vi "is hit.vi"(1 "Board with rocks":u32[][](array[numeric]), 2 "next row":i32, 3 "next column":i32, 4 "next orientation":i32) -> (0 "is hit":bool)   [LabVIEW 2019]
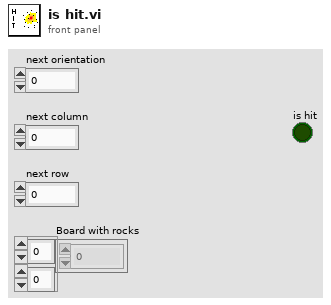
[diagram p1: front panel]
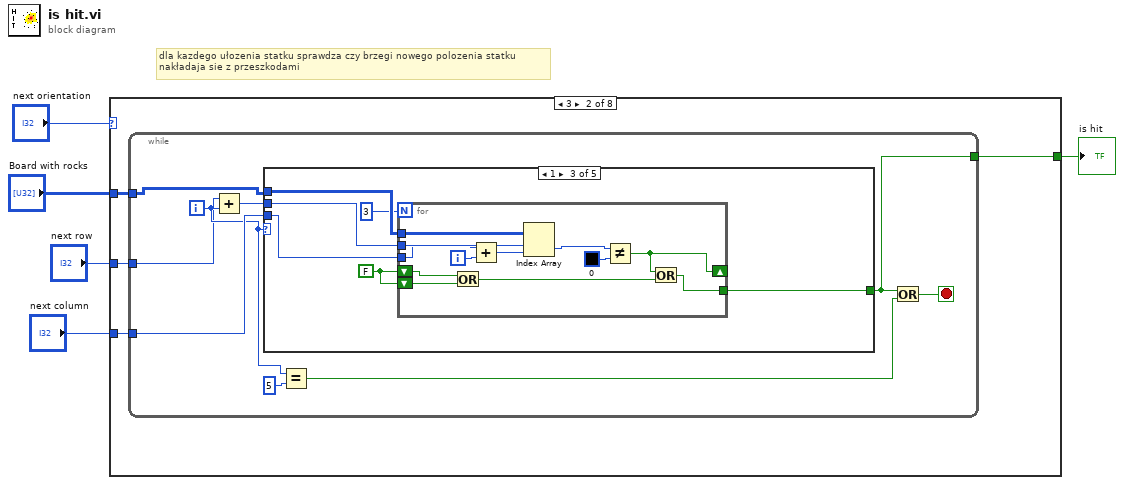
[diagram p0: block diagram]
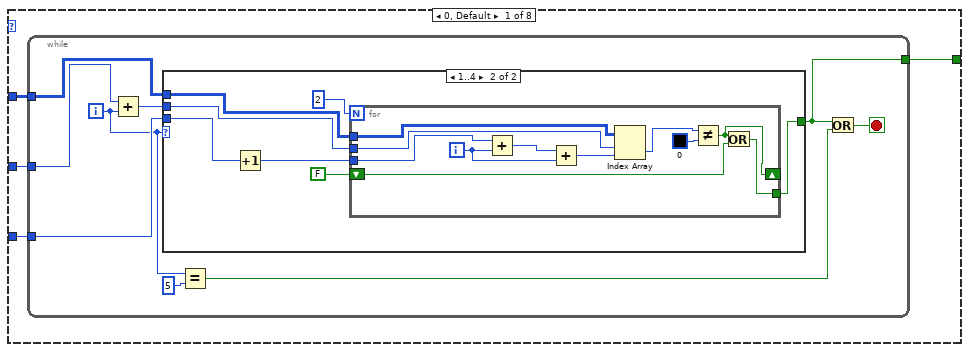
[diagram p2: hidden frame]
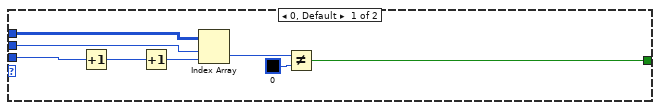
[diagram p3: hidden frame]
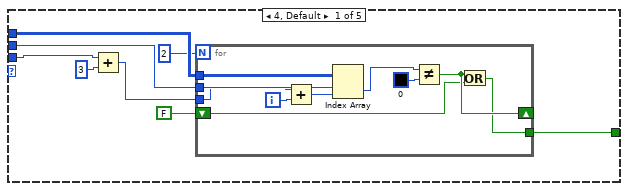
[diagram p4: hidden frame]
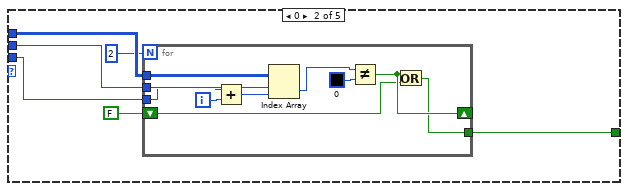
[diagram p5: hidden frame]
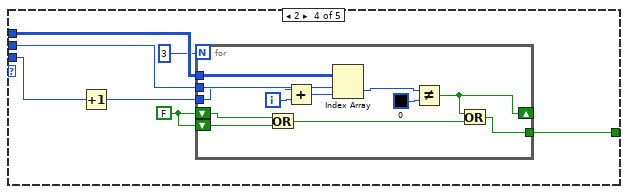
[diagram p6: hidden frame]
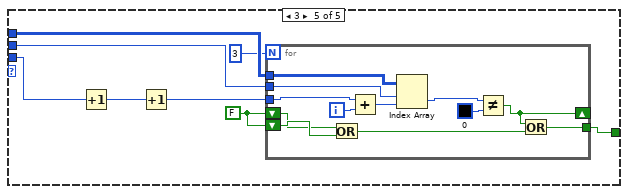
[diagram p7: hidden frame]
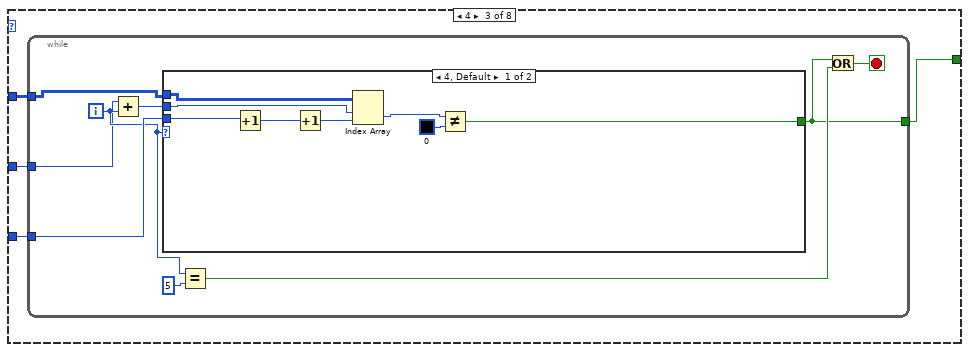
[diagram p8: hidden frame]
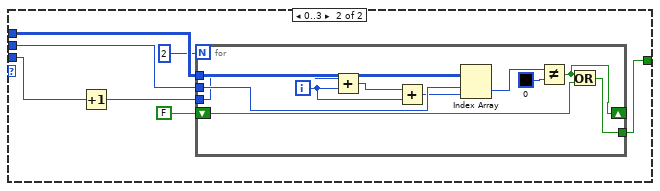
[diagram p9: hidden frame]
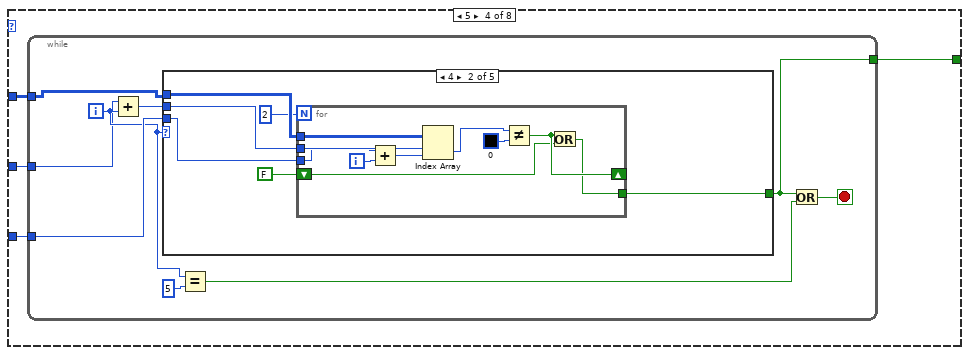
[diagram p10: hidden frame]
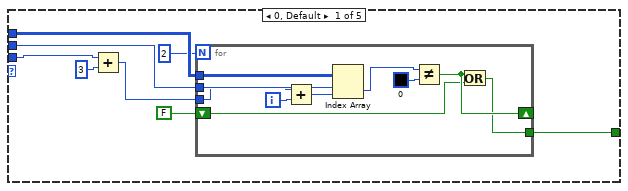
[diagram p11: hidden frame]
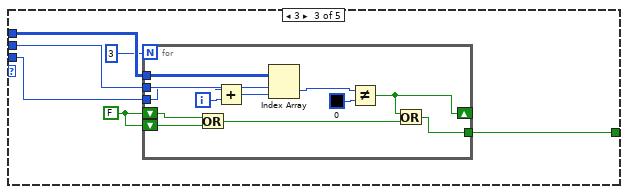
[diagram p12: hidden frame]
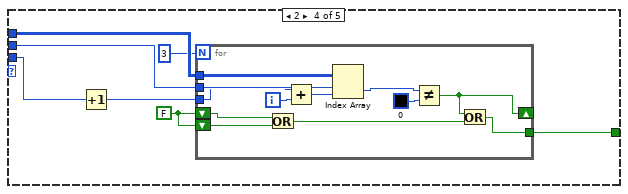
[diagram p13: hidden frame]
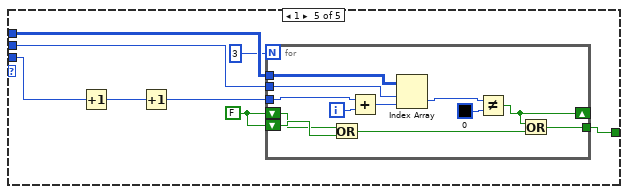
[diagram p14: hidden frame]
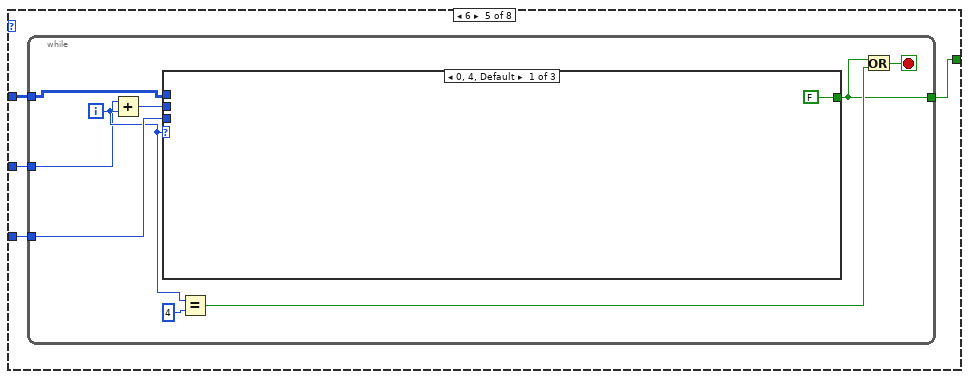
[diagram p15: hidden frame]
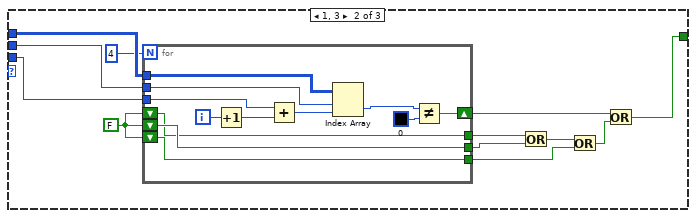
[diagram p16: hidden frame]
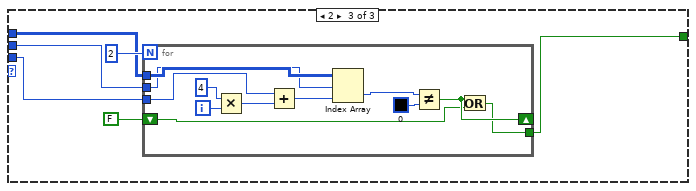
[diagram p17: hidden frame]
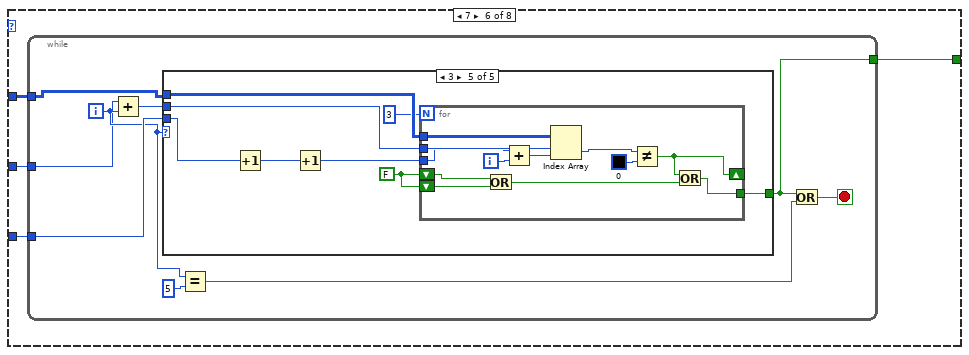
[diagram p18: hidden frame]
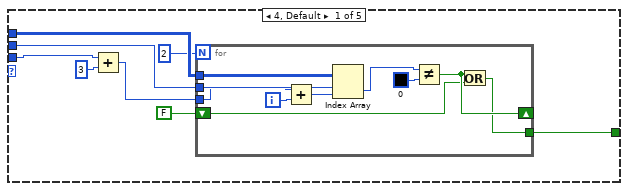
[diagram p19: hidden frame]
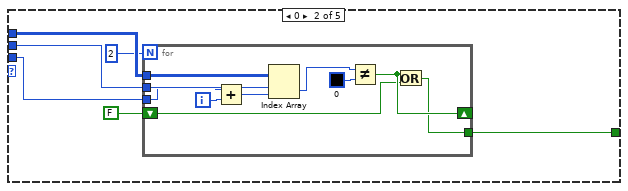
[diagram p20: hidden frame]
diagram:
  # "dla kazdego ułozenia statku sprawdza czy brzegi nowego polozenia statku \nnakładaja sie z przeszkodami"
  n1 = case shown="3" "next orientation" {
    tunnel: "next column" -> [w7 w46 w150 w189 w293 w349 w455 w557]
    tunnel: "next row" -> [w8 w47 w151 w190 w294 w350 w454 w558]
    tunnel: "Board with rocks" -> [w9 w48 w152 w191 w295 w351 w453 w559]
    tunnel: [w6 w45 w149 w188 w292 w348 w452 w556] -> w1
    frame 0, Default {
      n2 = while {
        tunnel: [w13] -> w6
        tunnel: w9 -> [w18]
        tunnel: w8 -> [w10]
        tunnel: w7 -> [w14]
        i -> [w12]
        stop <- w15 stop-if-true
        n3 = Add(x=w10, y=w12) -> (x+y=w11:i32)
        n4 = case shown="1..4" w12 {
          tunnel: w18 -> [w26 w33]
          tunnel: w11 -> [w25 w28]
          tunnel: w14 -> [w20 w30]
          tunnel: [w22 w27] -> w13
          frame 0, Default {
            n5 = Increment(x=w20) -> (x+1=w19:i32)
            n6 = Increment(x=w19) -> (x+1=w24:i32)
            n7 = Index Array(array=w26, index (row)=w25, index (col)=w24) -> (element=w21:u32)
            n8 = Not Equal?(x=w21, y=u32 0 ("Color Box")) -> (x != y?=w22:bool)
          }
          frame 1..4 {
            n9 = Increment(x=w30) -> (x+1=w29:i32)
            n10 = for {
              N: 2 -> [_]
              tunnel: w33 -> [w43]
              tunnel: w28 -> [w42]
              tunnel: w29 -> [w41]
              shift-right: [w36] -> _
              shift-left: FALSE -> [w35]
              tunnel: [w34] -> w27
              i -> [w38]
              n11 = Add(x=w41, y=w38) -> (x+y=w39:i32)
              n12 = Add(x=w39, y=w38) -> (x+y=w37:i32)
              n13 = Index Array(array=w43, index (row)=w42, index (col)=w37) -> (element=w40:u32)
              n14 = Not Equal?(x=w40, y=u32 0 ("Color Box")) -> (x != y?=w36:bool)
              n15 = Or(x=w36, y=w35) -> (x .or. y?=w34:bool)
            }
          }
        }
        n16 = Equal?(x=w12, y=5) -> (x = y?=w16:bool)
        n17 = Or(x=w13, y=w16) -> (x .or. y?=w15:bool)
      }
    }
    frame 3 {
      n18 = while {
        tunnel: [w52] -> w45
        tunnel: w48 -> [w57]
        tunnel: w47 -> [w49]
        tunnel: w46 -> [w53]
        i -> [w51]
        stop <- w54 stop-if-true
        n19 = Add(x=w49, y=w51) -> (x+y=w50:i32)
        n20 = case shown="1" w51 {
          tunnel: w57 -> [w65 w81 w97 w116 w136]
          tunnel: w50 -> [w62 w78 w95 w114 w134]
          tunnel: w53 -> [w60 w76 w93 w110 w131]
          tunnel: [w61 w77 w94 w113 w133] -> w52
          frame 4, Default {
            n21 = Add(x=w60, y=3) -> (x+y=w58:i32)
            n22 = for {
              N: 2 -> [_]
              tunnel: w65 -> [w74]
              tunnel: w62 -> [w73]
              tunnel: w58 -> [w72]
              shift-right: [w70] -> _
              shift-left: FALSE -> [w69]
              tunnel: [w68] -> w61
              i -> [w67]
              n23 = Add(x=w72, y=w67) -> (x+y=w66:i32)
              n24 = Index Array(array=w74, index (row)=w73, index (col)=w66) -> (element=w71:u32)
              n25 = Not Equal?(x=w71, y=u32 0 ("Color Box")) -> (x != y?=w70:bool)
              n26 = Or(x=w70, y=w69) -> (x .or. y?=w68:bool)
            }
          }
          frame 0 {
            n27 = for {
              N: 2 -> [_]
              tunnel: w81 -> [w90]
              tunnel: w78 -> [w89]
              tunnel: w76 -> [w88]
              shift-right: [w86] -> _
              shift-left: FALSE -> [w85]
              tunnel: [w84] -> w77
              i -> [w83]
              n28 = Add(x=w88, y=w83) -> (x+y=w82:i32)
              n29 = Index Array(array=w90, index (row)=w89, index (col)=w82) -> (element=w87:u32)
              n30 = Not Equal?(x=w87, y=u32 0 ("Color Box")) -> (x != y?=w86:bool)
              n31 = Or(x=w86, y=w85) -> (x .or. y?=w84:bool)
            }
          }
          frame 1 {
            w92 = FALSE
            n32 = for {
              N: 3 -> [_]
              tunnel: w97 -> [w108]
              tunnel: w95 -> [w107]
              tunnel: w93 -> [w106]
              shift-right: [w104] -> _
              shift-left: w92 -> [w99]
              tunnel: [w103] -> w94
              shift-left: w92 -> [w100]
              i -> [w102]
              n33 = Or(x=w99, y=w100) -> (x .or. y?=w98:bool)
              n34 = Add(x=w106, y=w102) -> (x+y=w101:i32)
              n35 = Index Array(array=w108, index (row)=w107, index (col)=w101) -> (element=w105:u32)
              n36 = Not Equal?(x=w105, y=u32 0 ("Color Box")) -> (x != y?=w104:bool)
              n37 = Or(x=w104, y=w98) -> (x .or. y?=w103:bool)
            }
          }
          frame 2 {
            w112 = FALSE
            n38 = Increment(x=w110) -> (x+1=w111:i32)
            n39 = for {
              N: 3 -> [_]
              tunnel: w116 -> [w127]
              tunnel: w114 -> [w126]
              tunnel: w111 -> [w125]
              shift-right: [w123] -> _
              shift-left: w112 -> [w118]
              tunnel: [w122] -> w113
              shift-left: w112 -> [w119]
              i -> [w121]
              n40 = Or(x=w118, y=w119) -> (x .or. y?=w117:bool)
              n41 = Add(x=w125, y=w121) -> (x+y=w120:i32)
              n42 = Index Array(array=w127, index (row)=w126, index (col)=w120) -> (element=w124:u32)
              n43 = Not Equal?(x=w124, y=u32 0 ("Color Box")) -> (x != y?=w123:bool)
              n44 = Or(x=w123, y=w117) -> (x .or. y?=w122:bool)
            }
          }
          frame 3 {
            w132 = FALSE
            n45 = Increment(x=w131) -> (x+1=w130:i32)
            n46 = Increment(x=w130) -> (x+1=w129:i32)
            n47 = for {
              N: 3 -> [_]
              tunnel: w136 -> [w147]
              tunnel: w134 -> [w146]
              tunnel: w129 -> [w145]
              shift-right: [w143] -> _
              shift-left: w132 -> [w138]
              tunnel: [w142] -> w133
              shift-left: w132 -> [w139]
              i -> [w141]
              n48 = Or(x=w138, y=w139) -> (x .or. y?=w137:bool)
              n49 = Add(x=w145, y=w141) -> (x+y=w140:i32)
              n50 = Index Array(array=w147, index (row)=w146, index (col)=w140) -> (element=w144:u32)
              n51 = Not Equal?(x=w144, y=u32 0 ("Color Box")) -> (x != y?=w143:bool)
              n52 = Or(x=w143, y=w137) -> (x .or. y?=w142:bool)
            }
          }
        }
        n53 = Equal?(x=w51, y=5) -> (x = y?=w55:bool)
        n54 = Or(x=w52, y=w55) -> (x .or. y?=w54:bool)
      }
    }
    frame 4 {
      n55 = while {
        tunnel: [w156] -> w149
        tunnel: w152 -> [w161]
        tunnel: w151 -> [w153]
        tunnel: w150 -> [w157]
        i -> [w155]
        stop <- w158 stop-if-true
        n56 = Add(x=w153, y=w155) -> (x+y=w154:i32)
        n57 = case shown="4, Default" w155 {
          tunnel: w161 -> [w169 w176]
          tunnel: w154 -> [w168 w171]
          tunnel: w157 -> [w163 w173]
          tunnel: [w165 w170] -> w156
          frame 4, Default {
            n58 = Increment(x=w163) -> (x+1=w162:i32)
            n59 = Increment(x=w162) -> (x+1=w167:i32)
            n60 = Index Array(array=w169, index (row)=w168, index (col)=w167) -> (element=w164:u32)
            n61 = Not Equal?(x=w164, y=u32 0 ("Color Box")) -> (x != y?=w165:bool)
          }
          frame 0..3 {
            n62 = Increment(x=w173) -> (x+1=w172:i32)
            n63 = for {
              N: 2 -> [_]
              tunnel: w176 -> [w186]
              tunnel: w171 -> [w185]
              tunnel: w172 -> [w184]
              shift-right: [w179] -> _
              shift-left: FALSE -> [w178]
              tunnel: [w177] -> w170
              i -> [w181]
              n64 = Add(x=w184, y=w181) -> (x+y=w182:i32)
              n65 = Add(x=w182, y=w181) -> (x+y=w180:i32)
              n66 = Index Array(array=w186, index (row)=w185, index (col)=w180) -> (element=w183:u32)
              n67 = Not Equal?(x=w183, y=u32 0 ("Color Box")) -> (x != y?=w179:bool)
              n68 = Or(x=w179, y=w178) -> (x .or. y?=w177:bool)
            }
          }
        }
        n69 = Equal?(x=w155, y=5) -> (x = y?=w159:bool)
        n70 = Or(x=w156, y=w159) -> (x .or. y?=w158:bool)
      }
    }
    frame 5 {
      n71 = while {
        tunnel: [w195] -> w188
        tunnel: w191 -> [w200]
        tunnel: w190 -> [w192]
        tunnel: w189 -> [w196]
        i -> [w194]
        stop <- w197 stop-if-true
        n72 = Add(x=w192, y=w194) -> (x+y=w193:i32)
        n73 = case shown="4" w194 {
          tunnel: w200 -> [w208 w224 w240 w259 w279]
          tunnel: w193 -> [w205 w221 w238 w257 w277]
          tunnel: w196 -> [w203 w219 w236 w253 w274]
          tunnel: [w204 w220 w237 w256 w276] -> w195
          frame 0, Default {
            n74 = Add(x=w203, y=3) -> (x+y=w201:i32)
            n75 = for {
              N: 2 -> [_]
              tunnel: w208 -> [w217]
              tunnel: w205 -> [w216]
              tunnel: w201 -> [w215]
              shift-right: [w213] -> _
              shift-left: FALSE -> [w212]
              tunnel: [w211] -> w204
              i -> [w210]
              n76 = Add(x=w215, y=w210) -> (x+y=w209:i32)
              n77 = Index Array(array=w217, index (row)=w216, index (col)=w209) -> (element=w214:u32)
              n78 = Not Equal?(x=w214, y=u32 0 ("Color Box")) -> (x != y?=w213:bool)
              n79 = Or(x=w213, y=w212) -> (x .or. y?=w211:bool)
            }
          }
          frame 4 {
            n80 = for {
              N: 2 -> [_]
              tunnel: w224 -> [w233]
              tunnel: w221 -> [w232]
              tunnel: w219 -> [w231]
              shift-right: [w229] -> _
              shift-left: FALSE -> [w228]
              tunnel: [w227] -> w220
              i -> [w226]
              n81 = Add(x=w231, y=w226) -> (x+y=w225:i32)
              n82 = Index Array(array=w233, index (row)=w232, index (col)=w225) -> (element=w230:u32)
              n83 = Not Equal?(x=w230, y=u32 0 ("Color Box")) -> (x != y?=w229:bool)
              n84 = Or(x=w229, y=w228) -> (x .or. y?=w227:bool)
            }
          }
          frame 3 {
            w235 = FALSE
            n85 = for {
              N: 3 -> [_]
              tunnel: w240 -> [w251]
              tunnel: w238 -> [w250]
              tunnel: w236 -> [w249]
              shift-right: [w247] -> _
              shift-left: w235 -> [w242]
              tunnel: [w246] -> w237
              shift-left: w235 -> [w243]
              i -> [w245]
              n86 = Or(x=w242, y=w243) -> (x .or. y?=w241:bool)
              n87 = Add(x=w249, y=w245) -> (x+y=w244:i32)
              n88 = Index Array(array=w251, index (row)=w250, index (col)=w244) -> (element=w248:u32)
              n89 = Not Equal?(x=w248, y=u32 0 ("Color Box")) -> (x != y?=w247:bool)
              n90 = Or(x=w247, y=w241) -> (x .or. y?=w246:bool)
            }
          }
          frame 2 {
            w255 = FALSE
            n91 = Increment(x=w253) -> (x+1=w254:i32)
            n92 = for {
              N: 3 -> [_]
              tunnel: w259 -> [w270]
              tunnel: w257 -> [w269]
              tunnel: w254 -> [w268]
              shift-right: [w266] -> _
              shift-left: w255 -> [w261]
              tunnel: [w265] -> w256
              shift-left: w255 -> [w262]
              i -> [w264]
              n93 = Or(x=w261, y=w262) -> (x .or. y?=w260:bool)
              n94 = Add(x=w268, y=w264) -> (x+y=w263:i32)
              n95 = Index Array(array=w270, index (row)=w269, index (col)=w263) -> (element=w267:u32)
              n96 = Not Equal?(x=w267, y=u32 0 ("Color Box")) -> (x != y?=w266:bool)
              n97 = Or(x=w266, y=w260) -> (x .or. y?=w265:bool)
            }
          }
          frame 1 {
            w275 = FALSE
            n98 = Increment(x=w274) -> (x+1=w273:i32)
            n99 = Increment(x=w273) -> (x+1=w272:i32)
            n100 = for {
              N: 3 -> [_]
              tunnel: w279 -> [w290]
              tunnel: w277 -> [w289]
              tunnel: w272 -> [w288]
              shift-right: [w286] -> _
              shift-left: w275 -> [w281]
              tunnel: [w285] -> w276
              shift-left: w275 -> [w282]
              i -> [w284]
              n101 = Or(x=w281, y=w282) -> (x .or. y?=w280:bool)
              n102 = Add(x=w288, y=w284) -> (x+y=w283:i32)
              n103 = Index Array(array=w290, index (row)=w289, index (col)=w283) -> (element=w287:u32)
              n104 = Not Equal?(x=w287, y=u32 0 ("Color Box")) -> (x != y?=w286:bool)
              n105 = Or(x=w286, y=w280) -> (x .or. y?=w285:bool)
            }
          }
        }
        n106 = Equal?(x=w194, y=5) -> (x = y?=w198:bool)
        n107 = Or(x=w195, y=w198) -> (x .or. y?=w197:bool)
      }
    }
    frame 6 {
      n108 = while {
        tunnel: [w299] -> w292
        tunnel: w295 -> [w304]
        tunnel: w294 -> [w296]
        tunnel: w293 -> [w300]
        i -> [w298]
        stop <- w301 stop-if-true
        n109 = Add(x=w296, y=w298) -> (x+y=w297:i32)
        n110 = case shown="0, 4, Default" w298 {
          tunnel: w304 -> [_ w317 w333]
          tunnel: w297 -> [_ w315 w332]
          tunnel: w300 -> [_ w314 w331]
          tunnel: [FALSE w307 w330] -> w299
          frame 0, 4, Default {
          }
          frame 1, 3 {
            w313 = FALSE
            n111 = for {
              N: 4 -> [_]
              tunnel: w317 -> [w328]
              tunnel: w315 -> [w327]
              tunnel: w314 -> [w326]
              shift-right: [w324] -> w309
              shift-left: w313 -> [w320]
              shift-left: w313 -> [w321]
              shift-left: w313 -> [w322]
              tunnel: [w322] -> w306
              tunnel: [w321] -> w311
              tunnel: [w320] -> w312
              i -> [w319]
              n112 = Increment(x=w319) -> (x+1=w318:i32)
              n113 = Add(x=w326, y=w318) -> (x+y=w323:i32)
              n114 = Index Array(array=w328, index (row)=w327, index (col)=w323) -> (element=w325:u32)
              n115 = Not Equal?(x=w325, y=u32 0 ("Color Box")) -> (x != y?=w324:bool)
            }
            n116 = Or(x=w312, y=w311) -> (x .or. y?=w310:bool)
            n117 = Or(x=w310, y=w306) -> (x .or. y?=w308:bool)
            n118 = Or(x=w309, y=w308) -> (x .or. y?=w307:bool)
          }
          frame 2 {
            n119 = for {
              N: 2 -> [_]
              tunnel: w333 -> [w346]
              tunnel: w332 -> [w345]
              tunnel: w331 -> [w338]
              shift-right: [w343] -> _
              shift-left: FALSE -> [w342]
              tunnel: [w341] -> w330
              i -> [w340]
              n120 = Multiply(x=4, y=w340) -> (x*y=w337:i32)
              n121 = Add(x=w338, y=w337) -> (x+y=w336:i32)
              n122 = Index Array(array=w346, index (row)=w345, index (col)=w336) -> (element=w344:u32)
              n123 = Not Equal?(x=w344, y=u32 0 ("Color Box")) -> (x != y?=w343:bool)
              n124 = Or(x=w343, y=w342) -> (x .or. y?=w341:bool)
            }
          }
        }
        n125 = Equal?(x=w298, y=4) -> (x = y?=w302:bool)
        n126 = Or(x=w299, y=w302) -> (x .or. y?=w301:bool)
      }
    }
    frame 7 {
      n127 = while {
        tunnel: [w355] -> w348
        tunnel: w351 -> [w360]
        tunnel: w350 -> [w352]
        tunnel: w349 -> [w356]
        i -> [w354]
        stop <- w357 stop-if-true
        n128 = Add(x=w352, y=w354) -> (x+y=w353:i32)
        n129 = case shown="3" w354 {
          tunnel: w360 -> [w368 w384 w400 w419 w439]
          tunnel: w353 -> [w365 w381 w398 w417 w437]
          tunnel: w356 -> [w363 w379 w396 w413 w434]
          tunnel: [w364 w380 w397 w416 w436] -> w355
          frame 4, Default {
            n130 = Add(x=w363, y=3) -> (x+y=w361:i32)
            n131 = for {
              N: 2 -> [_]
              tunnel: w368 -> [w377]
              tunnel: w365 -> [w376]
              tunnel: w361 -> [w375]
              shift-right: [w373] -> _
              shift-left: FALSE -> [w372]
              tunnel: [w371] -> w364
              i -> [w370]
              n132 = Add(x=w375, y=w370) -> (x+y=w369:i32)
              n133 = Index Array(array=w377, index (row)=w376, index (col)=w369) -> (element=w374:u32)
              n134 = Not Equal?(x=w374, y=u32 0 ("Color Box")) -> (x != y?=w373:bool)
              n135 = Or(x=w373, y=w372) -> (x .or. y?=w371:bool)
            }
          }
          frame 0 {
            n136 = for {
              N: 2 -> [_]
              tunnel: w384 -> [w393]
              tunnel: w381 -> [w392]
              tunnel: w379 -> [w391]
              shift-right: [w389] -> _
              shift-left: FALSE -> [w388]
              tunnel: [w387] -> w380
              i -> [w386]
              n137 = Add(x=w391, y=w386) -> (x+y=w385:i32)
              n138 = Index Array(array=w393, index (row)=w392, index (col)=w385) -> (element=w390:u32)
              n139 = Not Equal?(x=w390, y=u32 0 ("Color Box")) -> (x != y?=w389:bool)
              n140 = Or(x=w389, y=w388) -> (x .or. y?=w387:bool)
            }
          }
          frame 1 {
            w395 = FALSE
            n141 = for {
              N: 3 -> [_]
              tunnel: w400 -> [w411]
              tunnel: w398 -> [w410]
              tunnel: w396 -> [w409]
              shift-right: [w407] -> _
              shift-left: w395 -> [w402]
              tunnel: [w406] -> w397
              shift-left: w395 -> [w403]
              i -> [w405]
              n142 = Or(x=w402, y=w403) -> (x .or. y?=w401:bool)
              n143 = Add(x=w409, y=w405) -> (x+y=w404:i32)
              n144 = Index Array(array=w411, index (row)=w410, index (col)=w404) -> (element=w408:u32)
              n145 = Not Equal?(x=w408, y=u32 0 ("Color Box")) -> (x != y?=w407:bool)
              n146 = Or(x=w407, y=w401) -> (x .or. y?=w406:bool)
            }
          }
          frame 2 {
            w415 = FALSE
            n147 = Increment(x=w413) -> (x+1=w414:i32)
            n148 = for {
              N: 3 -> [_]
              tunnel: w419 -> [w430]
              tunnel: w417 -> [w429]
              tunnel: w414 -> [w428]
              shift-right: [w426] -> _
              shift-left: w415 -> [w421]
              tunnel: [w425] -> w416
              shift-left: w415 -> [w422]
              i -> [w424]
              n149 = Or(x=w421, y=w422) -> (x .or. y?=w420:bool)
              n150 = Add(x=w428, y=w424) -> (x+y=w423:i32)
              n151 = Index Array(array=w430, index (row)=w429, index (col)=w423) -> (element=w427:u32)
              n152 = Not Equal?(x=w427, y=u32 0 ("Color Box")) -> (x != y?=w426:bool)
              n153 = Or(x=w426, y=w420) -> (x .or. y?=w425:bool)
            }
          }
          frame 3 {
            w435 = FALSE
            n154 = Increment(x=w434) -> (x+1=w433:i32)
            n155 = Increment(x=w433) -> (x+1=w432:i32)
            n156 = for {
              N: 3 -> [_]
              tunnel: w439 -> [w450]
              tunnel: w437 -> [w449]
              tunnel: w432 -> [w448]
              shift-right: [w446] -> _
              shift-left: w435 -> [w441]
              tunnel: [w445] -> w436
              shift-left: w435 -> [w442]
              i -> [w444]
              n157 = Or(x=w441, y=w442) -> (x .or. y?=w440:bool)
              n158 = Add(x=w448, y=w444) -> (x+y=w443:i32)
              n159 = Index Array(array=w450, index (row)=w449, index (col)=w443) -> (element=w447:u32)
              n160 = Not Equal?(x=w447, y=u32 0 ("Color Box")) -> (x != y?=w446:bool)
              n161 = Or(x=w446, y=w440) -> (x .or. y?=w445:bool)
            }
          }
        }
        n162 = Equal?(x=w354, y=5) -> (x = y?=w358:bool)
        n163 = Or(x=w355, y=w358) -> (x .or. y?=w357:bool)
      }
    }
    frame 1 {
      n164 = while {
        tunnel: [w459] -> w452
        tunnel: w453 -> [w464]
        tunnel: w454 -> [w456]
        tunnel: w455 -> [w460]
        i -> [w458]
        stop <- w461 stop-if-true
        n165 = Add(x=w456, y=w458) -> (x+y=w457:i32)
        n166 = case shown="4" w458 {
          tunnel: w464 -> [w472 w488 w504 w523 w543]
          tunnel: w457 -> [w469 w485 w502 w521 w541]
          tunnel: w460 -> [w467 w483 w500 w517 w538]
          tunnel: [w468 w484 w501 w520 w540] -> w459
          frame 0, Default {
            n167 = Add(x=w467, y=3) -> (x+y=w465:i32)
            n168 = for {
              N: 2 -> [_]
              tunnel: w472 -> [w481]
              tunnel: w469 -> [w480]
              tunnel: w465 -> [w479]
              shift-right: [w477] -> _
              shift-left: FALSE -> [w476]
              tunnel: [w475] -> w468
              i -> [w474]
              n169 = Add(x=w479, y=w474) -> (x+y=w473:i32)
              n170 = Index Array(array=w481, index (row)=w480, index (col)=w473) -> (element=w478:u32)
              n171 = Not Equal?(x=w478, y=u32 0 ("Color Box")) -> (x != y?=w477:bool)
              n172 = Or(x=w477, y=w476) -> (x .or. y?=w475:bool)
            }
          }
          frame 4 {
            n173 = for {
              N: 2 -> [_]
              tunnel: w488 -> [w497]
              tunnel: w485 -> [w496]
              tunnel: w483 -> [w495]
              shift-right: [w493] -> _
              shift-left: FALSE -> [w492]
              tunnel: [w491] -> w484
              i -> [w490]
              n174 = Add(x=w495, y=w490) -> (x+y=w489:i32)
              n175 = Index Array(array=w497, index (row)=w496, index (col)=w489) -> (element=w494:u32)
              n176 = Not Equal?(x=w494, y=u32 0 ("Color Box")) -> (x != y?=w493:bool)
              n177 = Or(x=w493, y=w492) -> (x .or. y?=w491:bool)
            }
          }
          frame 3 {
            w499 = FALSE
            n178 = for {
              N: 3 -> [_]
              tunnel: w504 -> [w515]
              tunnel: w502 -> [w514]
              tunnel: w500 -> [w513]
              shift-right: [w511] -> _
              shift-left: w499 -> [w506]
              tunnel: [w510] -> w501
              shift-left: w499 -> [w507]
              i -> [w509]
              n179 = Or(x=w506, y=w507) -> (x .or. y?=w505:bool)
              n180 = Add(x=w513, y=w509) -> (x+y=w508:i32)
              n181 = Index Array(array=w515, index (row)=w514, index (col)=w508) -> (element=w512:u32)
              n182 = Not Equal?(x=w512, y=u32 0 ("Color Box")) -> (x != y?=w511:bool)
              n183 = Or(x=w511, y=w505) -> (x .or. y?=w510:bool)
            }
          }
          frame 2 {
            w519 = FALSE
            n184 = Increment(x=w517) -> (x+1=w518:i32)
            n185 = for {
              N: 3 -> [_]
              tunnel: w523 -> [w534]
              tunnel: w521 -> [w533]
              tunnel: w518 -> [w532]
              shift-right: [w530] -> _
              shift-left: w519 -> [w525]
              tunnel: [w529] -> w520
              shift-left: w519 -> [w526]
              i -> [w528]
              n186 = Or(x=w525, y=w526) -> (x .or. y?=w524:bool)
              n187 = Add(x=w532, y=w528) -> (x+y=w527:i32)
              n188 = Index Array(array=w534, index (row)=w533, index (col)=w527) -> (element=w531:u32)
              n189 = Not Equal?(x=w531, y=u32 0 ("Color Box")) -> (x != y?=w530:bool)
              n190 = Or(x=w530, y=w524) -> (x .or. y?=w529:bool)
            }
          }
          frame 1 {
            w539 = FALSE
            n191 = Increment(x=w538) -> (x+1=w537:i32)
            n192 = Increment(x=w537) -> (x+1=w536:i32)
            n193 = for {
              N: 3 -> [_]
              tunnel: w543 -> [w554]
              tunnel: w541 -> [w553]
              tunnel: w536 -> [w552]
              shift-right: [w550] -> _
              shift-left: w539 -> [w545]
              tunnel: [w549] -> w540
              shift-left: w539 -> [w546]
              i -> [w548]
              n194 = Or(x=w545, y=w546) -> (x .or. y?=w544:bool)
              n195 = Add(x=w552, y=w548) -> (x+y=w547:i32)
              n196 = Index Array(array=w554, index (row)=w553, index (col)=w547) -> (element=w551:u32)
              n197 = Not Equal?(x=w551, y=u32 0 ("Color Box")) -> (x != y?=w550:bool)
              n198 = Or(x=w550, y=w544) -> (x .or. y?=w549:bool)
            }
          }
        }
        n199 = Equal?(x=w458, y=5) -> (x = y?=w462:bool)
        n200 = Or(x=w459, y=w462) -> (x .or. y?=w461:bool)
      }
    }
    frame 2 {
      n201 = while {
        tunnel: [w563] -> w556
        tunnel: w559 -> [w568]
        tunnel: w558 -> [w560]
        tunnel: w557 -> [w564]
        i -> [w562]
        stop <- w565 stop-if-true
        n202 = Add(x=w560, y=w562) -> (x+y=w561:i32)
        n203 = case shown="0, 4, Default" w562 {
          tunnel: w568 -> [_ w581 w596]
          tunnel: w561 -> [_ w579 w595]
          tunnel: w564 -> [_ w578 w594]
          tunnel: [FALSE w571 w593] -> w563
          frame 0, 4, Default {
          }
          frame 1, 3 {
            w577 = FALSE
            n204 = for {
              N: 4 -> [_]
              tunnel: w581 -> [w591]
              tunnel: w579 -> [w590]
              tunnel: w578 -> [w589]
              shift-right: [w586] -> w573
              shift-left: w577 -> [w582]
              shift-left: w577 -> [w583]
              shift-left: w577 -> [w584]
              tunnel: [w584] -> w570
              tunnel: [w583] -> w575
              tunnel: [w582] -> w576
              i -> [w587]
              n205 = Add(x=w589, y=w587) -> (x+y=w585:i32)
              n206 = Index Array(array=w591, index (row)=w590, index (col)=w585) -> (element=w588:u32)
              n207 = Not Equal?(x=w588, y=u32 0 ("Color Box")) -> (x != y?=w586:bool)
            }
            n208 = Or(x=w576, y=w575) -> (x .or. y?=w574:bool)
            n209 = Or(x=w574, y=w570) -> (x .or. y?=w572:bool)
            n210 = Or(x=w573, y=w572) -> (x .or. y?=w571:bool)
          }
          frame 2 {
            n211 = for {
              N: 2 -> [_]
              tunnel: w596 -> [w609]
              tunnel: w595 -> [w608]
              tunnel: w594 -> [w601]
              shift-right: [w606] -> _
              shift-left: FALSE -> [w605]
              tunnel: [w604] -> w593
              i -> [w603]
              n212 = Multiply(x=4, y=w603) -> (x*y=w600:i32)
              n213 = Add(x=w601, y=w600) -> (x+y=w599:i32)
              n214 = Index Array(array=w609, index (row)=w608, index (col)=w599) -> (element=w607:u32)
              n215 = Not Equal?(x=w607, y=u32 0 ("Color Box")) -> (x != y?=w606:bool)
              n216 = Or(x=w606, y=w605) -> (x .or. y?=w604:bool)
            }
          }
        }
        n217 = Equal?(x=w562, y=4) -> (x = y?=w566:bool)
        n218 = Or(x=w563, y=w566) -> (x .or. y?=w565:bool)
      }
    }
  }
  "is hit" <- w1
